vi "Cipher to Number.vi"(8 "error in (no error)":errorcluster, 11 "Ciphers":i32[](array[numeric])) -> (0 "error out":errorcluster, 1 "Negative":bool, 3 "Number":i32)   [LabVIEW 2018, in "Resistance Value.lvlib"]
doc: "Converts an array of decimal digits into an integer number.\n\nThe VI receives the <b>Ciphers</b> array and constructs the corresponding integer value by processing each element sequentially.\n\nEach element of the array represents one decimal digit. The first element may be negative to indicate the sign of the resulting number. All subsequent elements must be in the range 0 to 9.\n\nThe VI returns the resulting integer through <b>Number</b> and indicates the detected sign through <b>Negative</b>.\n\nInvalid cipher values generate an error through <b>error out</b>."
uses:
  <vilib>/Utility/error.llb/Error Cluster From Error Code.vi
  <vilib>/ErrorRing/Error Ring.xnode
  Resistance Value.lvlib
panel:
  # "index = 0 -> LSD\nindex = 1 -> ....\n\nindex = n -> MSD"
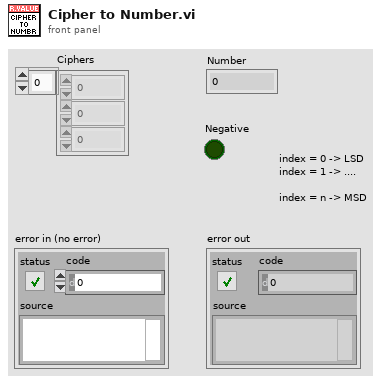
[diagram p1: front panel]
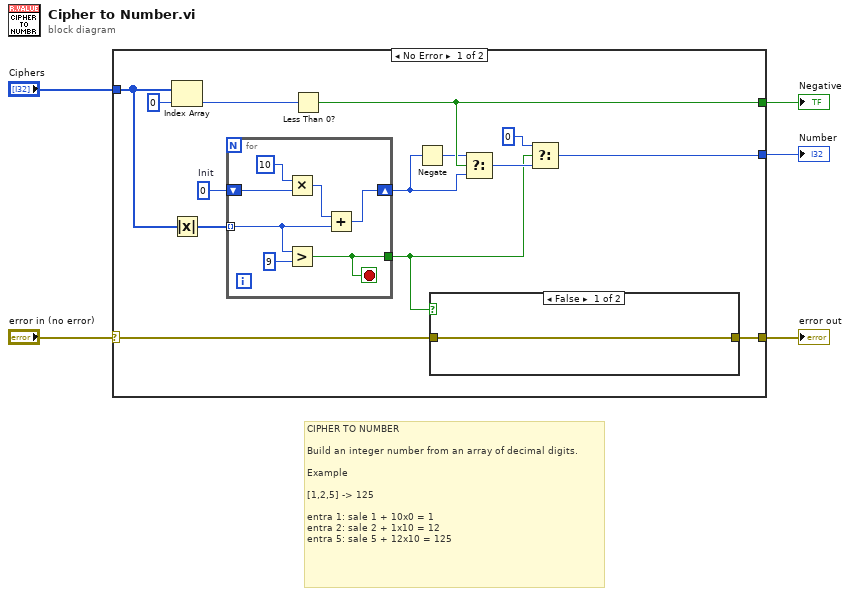
[diagram p0: block diagram]
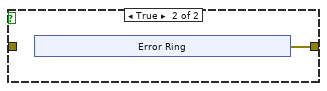
[diagram p2: hidden frame]
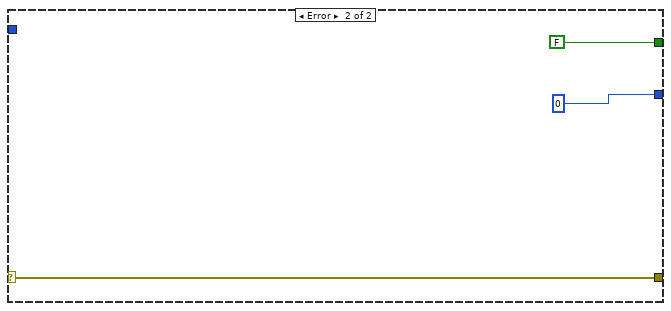
[diagram p3: hidden frame]
diagram:
  # "CIPHER TO NUMBER\n\nBuild an integer number from an array of decimal digits.\n\nExample\n\n[1,2,5] -> 125\n\nentra 1: sale 1 + 10x0 = 1\nentra 2: sale 2 + 1x10 = 12\nentra 5: sale 5 + 12x10 = 125"
  n1 = case shown="No Error" "error in (no error)" {
    selector: "error in (no error)" -> [w8 w36]
    tunnel: "Ciphers" -> [w18 _]
    tunnel: [w12 0 ("Init")] -> w4
    tunnel: [w11 FALSE] -> w3
    tunnel: [w9 w36] -> w2
    frame No Error {
      w16 = 0  # Init
      n2 = Index Array(array=w18, index=0) -> (element=w15:i32)
      n3 = Absolute Value(x=w18) -> (abs(x)=w17:i32[])
      n4 = for {
        tunnel: w17 -> [w29] mode=indexing
        shift-right: [w33] -> w7
        shift-left: w16 -> [w32]
        tunnel: [w27] -> w10
        stop <- w27 stop-if-true
        n5 = Multiply(x=10, y=w32) -> (x*y=w30:i32)
        n6 = Greater?(x=w29, y=9) -> (0:w27:bool)
        n7 = Add(x=w30, y=w29) -> (x+y=w33:i32)
      }
      n8 = Less Than 0?(x=w15) -> (x < 0?=w11:bool)
      n9 = Negate(x=w7) -> (-x=w6:i32)
      n10 = case shown="False" w10 {
        tunnel: [w20 w21] -> w9
        tunnel: w8 -> [w20 _]
        frame False {
        }
        frame True {
          n11 = xnode "Error Ring"() -> ("error out"=w21:errorcluster)
        }
      }
      n12 = Select(t=w6, s=w11, f=w7) -> (s? t:f=w14:i32)
      n13 = Select(t=0, s=w10, f=w14) -> (s? t:f=w12:i32)
    }
    frame Error {
    }
  }
  "Number" <- w4
  "Negative" <- w3
  "error out" <- w2
